vi "GetArrayElementClass.vi"(5 "Control in":refnum<class "Control.lvclass">, 6 "error in":errorcluster, 9 "PythonConverter_GUI in":refnum<class "PythonConverter_GUI.lvclass">) -> (0 "error out":errorcluster, 3 "PythonConverter_GUI out":refnum<class "PythonConverter_GUI.lvclass">, 4 "class":string)   [LabVIEW 2014, in "PythonConverter_GUI.lvclass"]
uses:
  PythonConverter_GUI.lvclass
  VI Interpreter/Classes/Control/Control.lvclass
  Parsing/ClassTypeTD.ctl
  PythonConverter_GUI.lvclass/PythonConverter_GUI.ctl
  VI Interpreter/Classes/Array/Array.lvclass
  Parsing/Python Functions.lvlib
  VI Interpreter/Classes/VI Interpreter/VI Interpreter.lvclass
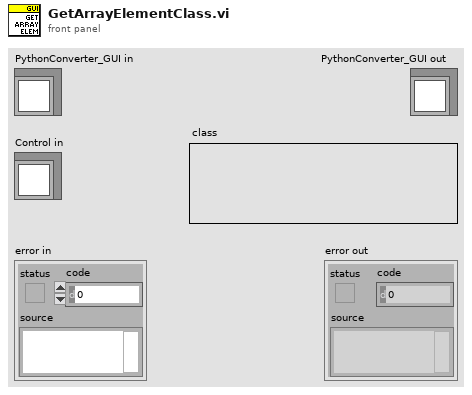
[diagram p1: front panel]
types:
  T1 = typedef "Python Functions.lvlib/ClassTypeTD.ctl" = enum16{"class", "function"}
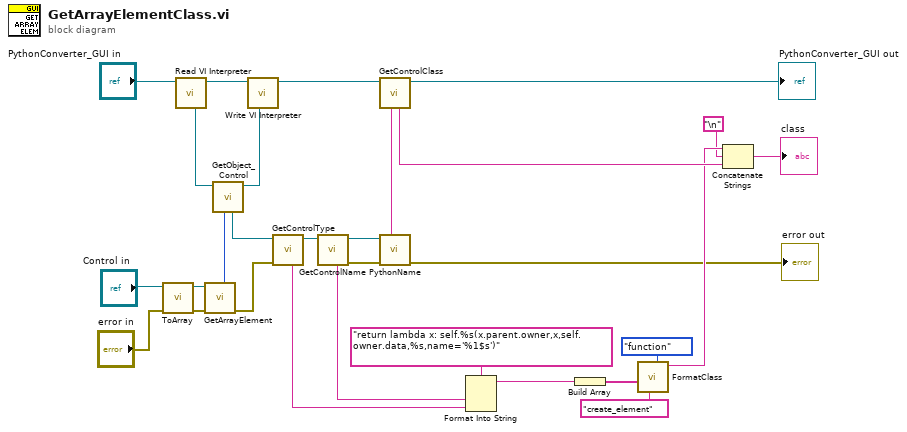
[diagram p0: block diagram]
diagram:
  n1 = call "ToArray.vi"("error in"="error in", "Generic in"="Control in") -> ("error out"=w28:errorcluster, "Array out"=w29:refnum<class "Array.lvclass">)  [unwired: 8 in]
  n2 = call "Read VI Interpreter.vi"("PythonConverter_GUI in"="PythonConverter_GUI in") -> ("PythonConverter_GUI out"=w18:refnum<class "PythonConverter_GUI.lvclass">, "VI Interpreter"=w21:refnum<class "VI Interpreter.lvclass">)  [unwired: 7 in]
  n3 = call "GetArrayElement.vi"("error in"=w28, "Array in"=w29) -> ("error out"=w10:errorcluster, "Array Element"=w20:i32)  [unwired: 5 in, 1 out]
  n4 = call "GetObject_Control.vi"("UID"=w20, "VI Interpreter in"=w21) -> ("VI Interpreter out"=w19:refnum<class "VI Interpreter.lvclass">, "control"=w11:refnum<class "Control.lvclass">)  [unwired: 4 in, 2 out]
  n5 = call "Write VI Interpreter.vi"("VI Interpreter"=w19, "PythonConverter_GUI in"=w18) -> ("PythonConverter_GUI out"=w13:refnum<class "PythonConverter_GUI.lvclass">)  [unwired: 7 in]
  n6 = call "GetControlType.vi"("error in"=w10, "Control in"=w11) -> ("Control out"=w12:refnum<class "Control.lvclass">, "type string"=w9:string)  [unwired: 7 in, 1 out]
  n7 = call "GetControlName.vi"("Control in"=w12) -> ("error out"=w15:errorcluster, "Control out"=w16:refnum<class "Control.lvclass">, "name"=w17:string)  [unwired: 6 in]
  n8 = call-dynamic "PythonName.vi"("error in"=w15, "GObject in"=w16) -> ("error out"=→"error out":errorcluster, "UID"=w14:string)  [unwired: 6 in, 2 out]
  n9 = call "GetControlClass.vi"("name"=w14, "PythonConverter_GUI in"=w13) -> ("PythonConverter_GUI out"=→"PythonConverter_GUI out":refnum<class "PythonConverter_GUI.lvclass">, "class"=w5:string)  [unwired: 5 in, 1 out]
  n10 = Format Into String(format string="return lambda x: self.%s(x.parent.owner,x,self.owner.data,%s,name='%1$s')", w17, w9) -> (resulting string=w8:string)  [unwired: 2 in, 1 out]
  n11 = Build Array(w8) -> (w7:string[])
  n12 = call "FormatClass.vi"("type"=ClassTypeTD."function", "name"="create_element", "body"=w7) -> ("python"=w4:string)  [unwired: 8 in]
  n13 = Concatenate Strings(w4, "\n", w5) -> (→"class":string)
